vi "Voorbeeld_Shift_Registervi.vi"() -> ()   [LabVIEW 2019]
panel:
  out "Waveform Chart":cluster{dbl, dbl}(graph)
  in  "stop":bool
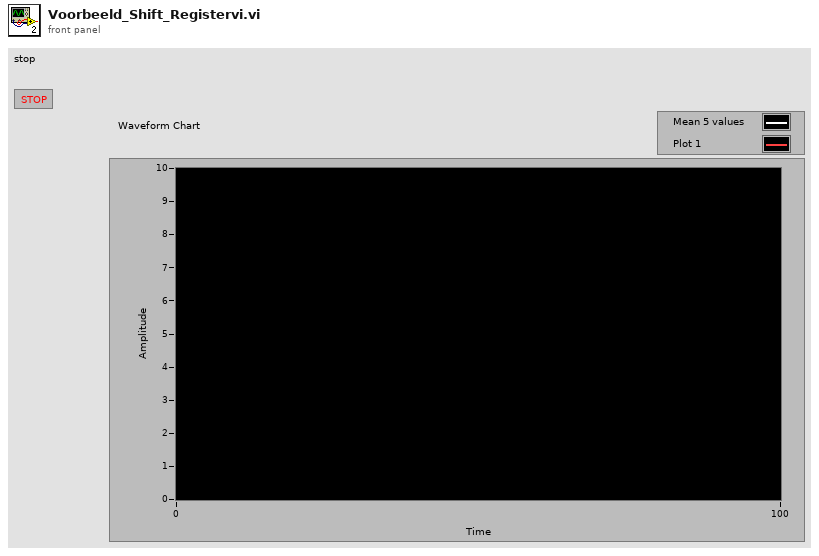
[diagram p1: front panel]
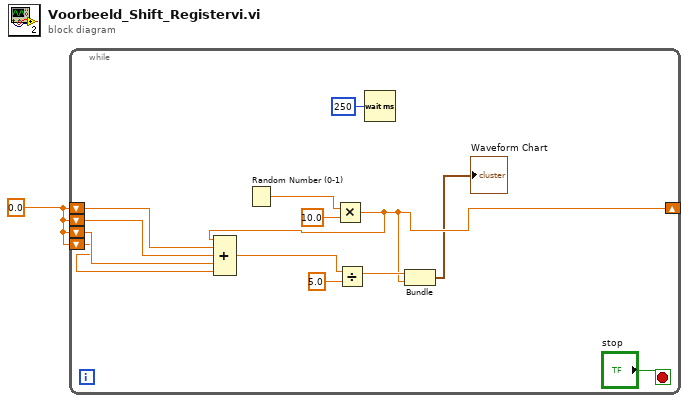
[diagram p0: block diagram]
diagram:
  w1 = 0.0
  n1 = while {
    shift-right: [w3] -> _
    shift-left: w1 -> [w10]
    shift-left: w1 -> [w9]
    shift-left: w1 -> [w8]
    shift-left: w1 -> [w7]
    stop <- "stop" stop-if-true
    n2 = Random Number (0-1)() -> (number: 0 to 1=w13:dbl)
    n3 = Multiply(x=w13, y=10.0) -> (x*y=w3:dbl)
    n4 = Compound Arithmetic op=ADD(w3, w10, w9, w8, w7) -> (w6:dbl)
    n5 = Divide(x=w6, y=5.0) -> (x/y=w4:dbl)
    n6 = Wait (ms)(milliseconds to wait=u32 250) -> ()  [unwired: 1 out]
    n7 = Bundle(w4, w3) -> (→"Waveform Chart":cluster{dbl, dbl})  [unwired: 1 in]
  }
